vi "HeartRateMonitor1.vi"() -> ()   [LabVIEW 2014]
uses:
  <vilib>/measure/mamon.llb/Waveform Peak Detection for N Chan.vi
  <vilib>/measure/NI_MAPro.lvlib
panel:
  out "Unfiltered Collector":dynamicdata(graph)
  in  "stop":bool
  out "BPM":dbl
  out "Frequency":dbl
  out "scalar":dbl
  out "Filtered Signal":dynamicdata(graph)
  out "Raw Signal":dynamicdata(graph)
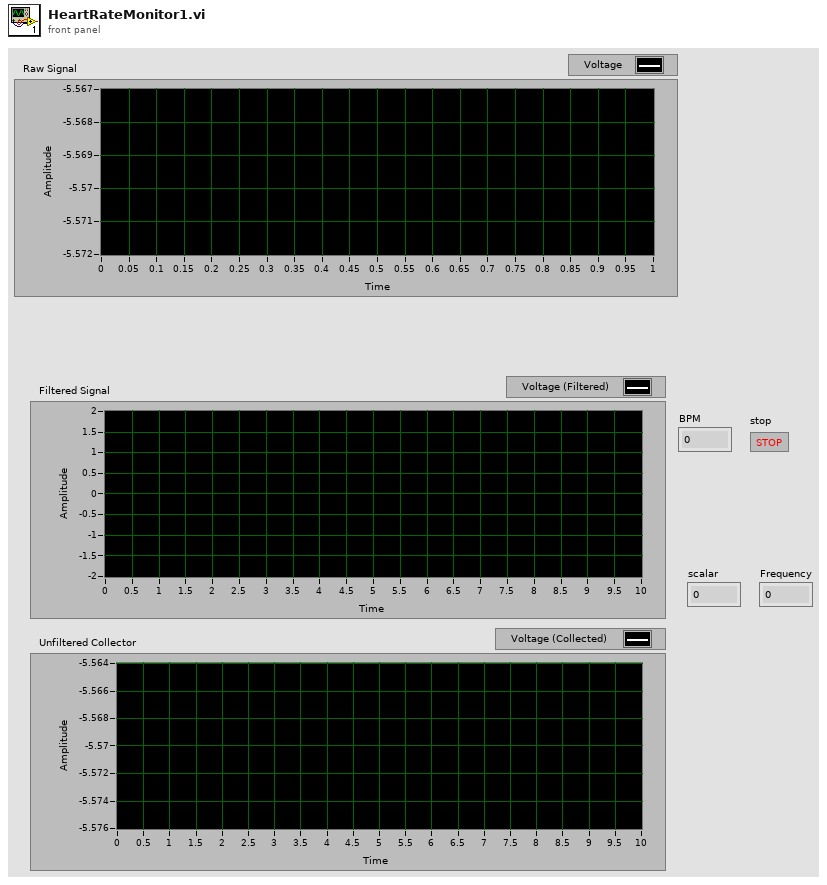
[diagram p1: front panel]
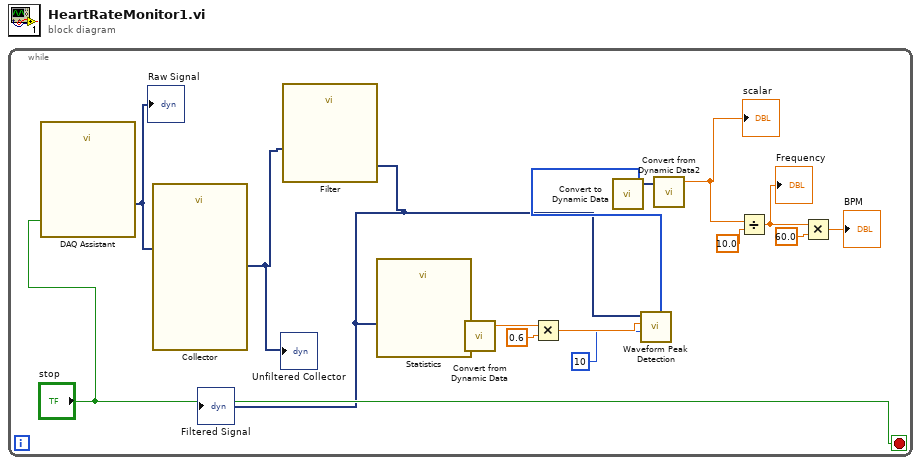
[diagram p0: block diagram]
diagram:
  n1 = while {
    stop <- "stop" stop-if-true
    n2 = call "DAQ Assistant"("stop (T)"="stop") -> ("data"=w3:dynamicdata)  [unwired: 16 in, 2 out]
    "Raw Signal" <- w3
    n3 = call "Collector"("Signals"=w3) -> ("Collected Signals"=w1:dynamicdata)  [unwired: 9 in, 1 out]
    "Unfiltered Collector" <- w1
    n4 = call "Filter"("Signal"=w1) -> ("Filtered Signal"=w2:dynamicdata)  [unwired: 9 in, 1 out]
    "Filtered Signal" <- w2
    n5 = call "Statistics"("Signals"=w2) -> ("Maximum"=w15:dynamicdata)  [unwired: 25 in, 1 out]
    n6 = call "Convert from Dynamic Data"("Dynamic Data Type"=w15) -> ("Scalar"=w14:dbl)  [unwired: 3 in]
    n7 = Multiply(x=w14, y=0.6) -> (x*y=w8:dbl)
    n8 = call-poly <vilib>:"Waveform Peak Detection.vi"("width"=10, "threshold"=w8, "Signals In"=w2) -> ("# found"=w6:i32[])  [unwired: 4 in, 4 out]
    n9 = call "Convert to Dynamic Data"("Array"=w6) -> ("Dynamic Data Type"=w5:dynamicdata)  [unwired: 3 in]
    n10 = call "Convert from Dynamic Data2"("Dynamic Data Type"=w5) -> ("Scalar"=w4:dbl)  [unwired: 3 in]
    "scalar" <- w4
    n11 = Divide(x=w4, y=10.0) -> (x/y=w12:dbl)
    "Frequency" <- w12
    n12 = Multiply(x=w12, y=60.0 ("Numeric")) -> (x*y=→"BPM":dbl)
  }
